vi "get_icons.vi"() -> ()   [LabVIEW 2017]
panel:
  out "Array":string[](array[string])
  out "Folders and Files":path[](array[path])
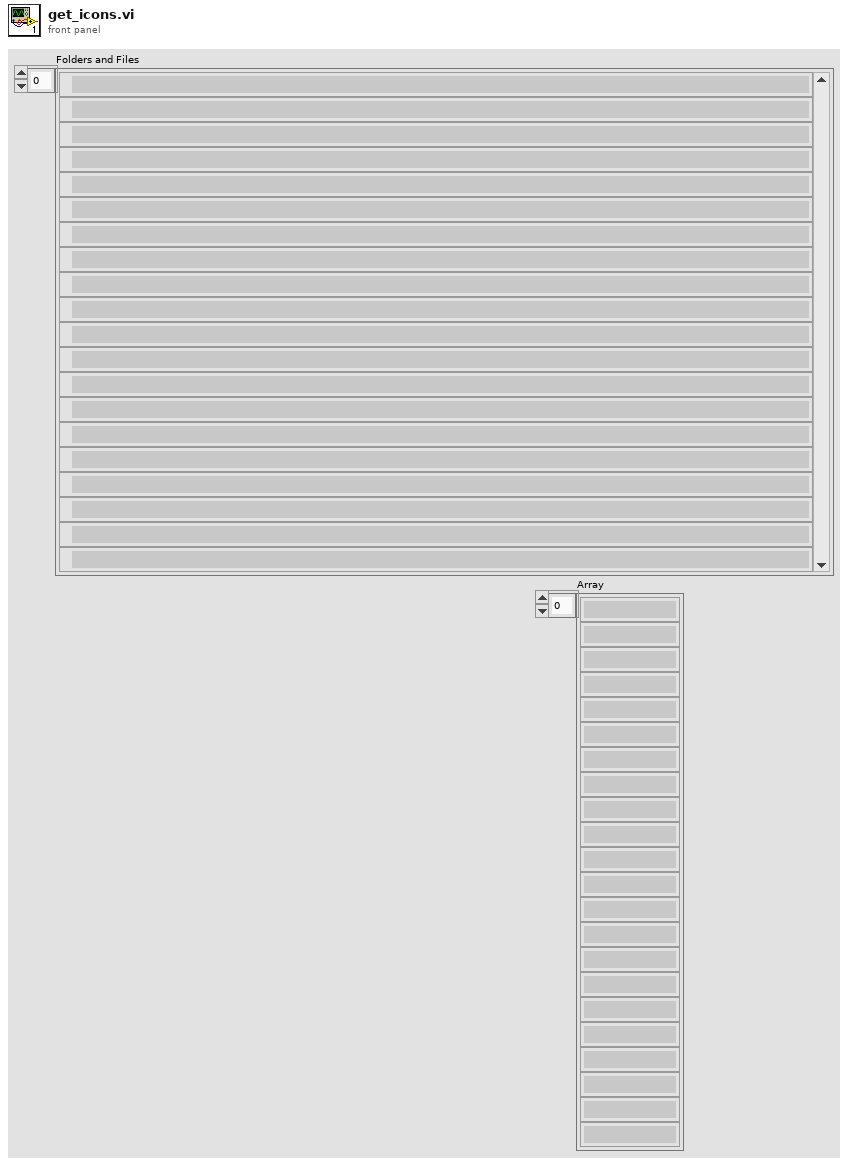
[diagram p1: front panel]
types:
  T1 = typedef "imagedata.ctl" = cluster{"image type":i32, "image depth":i32, "image":u8[], "mask":u8[], "colors":u32[], "Rectangle":cluster{"left":i16, "top":i16, "right":i16, "bottom":i16}}
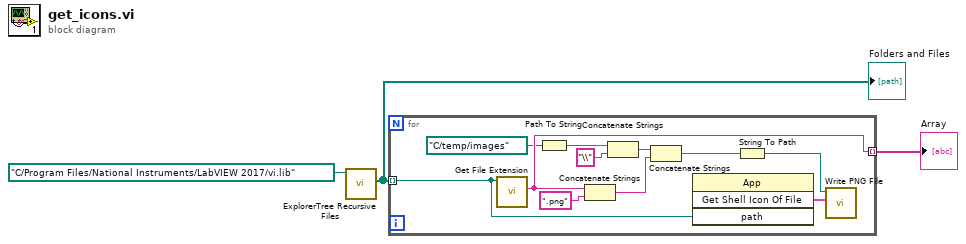
[diagram p0: block diagram]
diagram:
  n1 = call "ExplorerTree Recursive Files.vi"("Folder Path"=path "C:/Program Files/National Instruments/LabVIEW 2017/vi.lib" ("Path")) -> ("Folders and Files"=w2:path[])  [unwired: 7 in, 3 out]
  "Folders and Files" <- w2
  n2 = for {
    tunnel: w2 -> [w13] mode=indexing
    tunnel: [w12] -> w1 mode=indexing
    n3 = call <vilib>:"Get File Extension.vi"("file"=w13) -> ("lowercase file extension"=w12:string)  [unwired: 6 in, 4 out]
    n4 = Path To String(path=path "C:/temp/images" ("path to PNG file")) -> (string=w5:string)
    n5 = Concatenate Strings(w12, ".png" ("string")) -> (w9:string)
    n6 = Concatenate Strings(w5, "\\" ("string")) -> (w6:string)
    n7 = Concatenate Strings(w6, w9) -> (w8:string)
    n8 = invoke class="App" method="Get Shell Icon Of File"("path"=w13) -> ("GetShellIconOfFile"=w14:T1)  [unwired: 3 in, 3 out]
    n9 = String To Path(string=w8) -> (path=w7:path)
    n10 = call <vilib>:"Write PNG File.vi"("image data"=w14, "path to PNG file"=w7) -> ()  [unwired: 8 in, 2 out]
  }
  "Array" <- w1
